vi "Format Log String.vi"(11 "Log String In":string) -> (3 "Log String":string)   [LabVIEW 2015, in "Circular Error Log.lvclass"]
uses:
  Circular Error Log.lvclass
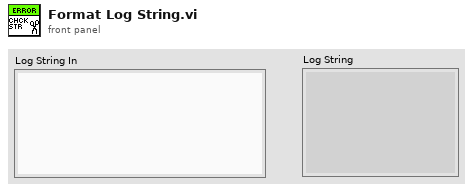
[diagram p1: front panel]
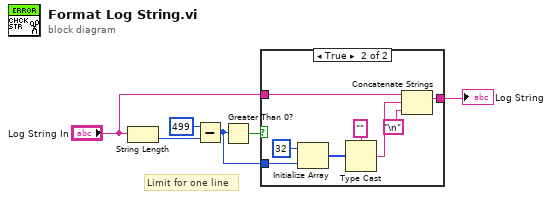
[diagram p0: block diagram]
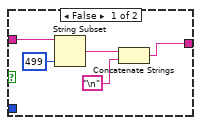
[diagram p2: hidden frame]
diagram:
  # "Limit for one line"
  n1 = String Length(string="Log String In") -> (length=w4:i32)
  n2 = Subtract(x=499 ("y"), y=w4) -> (x-y=w2:i32)
  n3 = Greater Than 0?(x=w2) -> (x > 0?=w3:bool)
  n4 = case shown="True" w3 {
    tunnel: "Log String In" -> [w11 w15]
    tunnel: [w8 w13] -> w1
    tunnel: w2 -> [_ w16]
    frame False {
      n5 = String Subset(string=w11, length (rest)=499 ("length (rest)")) -> (substring=w9:string)  [unwired: 1 in]
      n6 = Concatenate Strings(w9, "\n") -> (w8:string)
    }
    frame True {
      n7 = Initialize Array(u8 32 ("dimension size"), w16) -> (w18:u8[])
      n8 = Type Cast(type="", x=w18) -> (*(type *) &x=w14:string)
      n9 = Concatenate Strings(w15, w14, "\n") -> (w13:string)
    }
  }
  "Log String" <- w1
